vi "M Water Cells 90.vi"(11 "EV3 in":T1) -> (3 "EV3 out":T1)   [LabVIEW 2016]
uses:
  <vilib>/NXT/Subs/LVHSConnector.ctl
  <vilib>/NXT/LegoClasses/BrickReference/BrickReference.lvclass
  <vilib>/NXT/Dual Mode Library/Waits/Wait_Num.vi
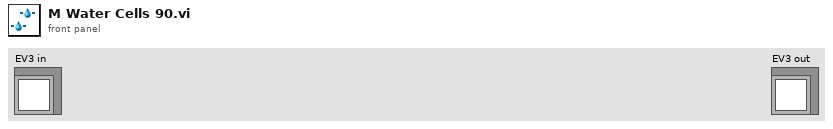
[diagram p1: front panel]
types:
  T1 = typedef "LVHSConnector.ctl" = refnum<class "BrickReference.lvclass">
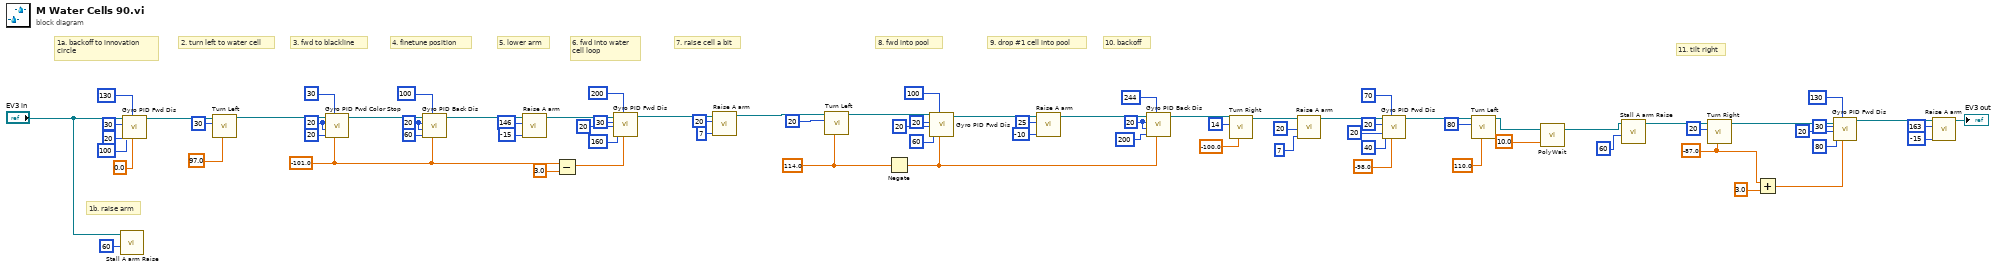
[diagram p0: block diagram]
diagram:
  w34 = sgl 114.0 ("Turning angle")
  w24 = sgl -87.0 ("Turning angle")
  w44 = 20 ("Max. speed")
  w63 = 20 ("Max. speed")
  w41 = sgl -101.0 ("Target angle")
  w67 = 20 ("Max. speed")
  # "11. tilt right"
  # "10. backoff"
  # "8. fwd into pool"
  # "6. fwd into water\ncell loop"
  # "4. finetune position"
  # "3. fwd to blackline"
  # "1b. raise arm"
  # "9. drop #1 cell into pool"
  # "7. raise cell a bit"
  # "5. lower arm"
  # "2. turn left to water cell"
  # "1a. backoff to innovation\ncircle"
  n1 = call "Stall A arm Raise.vi"("Power"=i8 60, "NXT/EV3"="EV3 in") -> ()  [unwired: 9 in, 1 out]
  n2 = call "Gyro PID Fwd Dis.vi"("Target angle"=sgl 0.0, "Threshold to stop"=130, "Threshold to slow"=100, "Min. speed"=20, "Max. speed"=30, "EV3 in"="EV3 in") -> ("EV3 out"=w76:T1)  [unwired: 5 in]
  n3 = call "Turn Left.vi"("Turning angle"=sgl 97.0, "Motor B (right)"=i8 30, "EV3 in"=w76) -> ("EV3 out"=w69:T1)  [unwired: 8 in]
  n4 = call "Gyro PID Fwd Color Stop.vi"("Target angle"=w41, "Threshold to Color"=30, "Threshold to slow"=20, "Min. speed"=w67, "Max. speed"=w67, "EV3 in"=w69) -> ("EV3 out"=w65:T1)  [unwired: 5 in]
  n5 = call "Gyro PID Back Dis.vi"("Target angle"=w41, "Threshold to stop"=100, "Threshold to slow"=60, "Min. speed"=w63, "Max. speed"=w63, "EV3 in"=w65) -> ("EV3 out"=w61:T1)  [unwired: 5 in]
  n6 = call "Raise A arm.vi"("Power"=i8 -15, "Rotation"=146, "EV3 in"=w61) -> ("EV3 out"=w60:T1)  [unwired: 8 in]
  n7 = Subtract(x=w41, y=sgl 3.0) -> (x-y=w39:sgl)
  n8 = call "Gyro PID Fwd Dis.vi"("Target angle"=w39, "Threshold to stop"=200, "Threshold to slow"=160, "Min. speed"=20, "Max. speed"=30, "EV3 in"=w60) -> ("EV3 out"=w55:T1)  [unwired: 5 in]
  n9 = call "Raise A arm.vi"("Power"=i8 7, "Rotation"=20, "EV3 in"=w55) -> ("EV3 out"=w37:T1)  [unwired: 8 in]
  n10 = call "Turn Left.vi"("Turning angle"=w34, "Motor B (right)"=i8 20, "EV3 in"=w37) -> ("EV3 out"=w36:T1)  [unwired: 8 in]
  n11 = Negate(x=w34) -> (-x=w33:sgl)
  n12 = call "Gyro PID Fwd Dis.vi"("Target angle"=w33, "Threshold to stop"=100, "Threshold to slow"=60, "Min. speed"=20, "Max. speed"=20, "EV3 in"=w36) -> ("EV3 out"=w47:T1)  [unwired: 5 in]
  n13 = call "Raise A arm.vi"("Power"=i8 -10, "Rotation"=25, "EV3 in"=w47) -> ("EV3 out"=w42:T1)  [unwired: 8 in]
  n14 = call "Gyro PID Back Dis.vi"("Target angle"=w33, "Threshold to stop"=244, "Threshold to slow"=200, "Min. speed"=w44, "Max. speed"=w44, "EV3 in"=w42) -> ("EV3 out"=w15:T1)  [unwired: 5 in]
  n15 = call "Turn Right.vi"("Turning angle"=sgl -100.0, "Motor B (right)"=i8 14, "EV3 in"=w15) -> ("EV3 out"=w13:T1)  [unwired: 8 in]
  n16 = call "Raise A arm.vi"("Power"=i8 7, "Rotation"=20, "EV3 in"=w13) -> ("EV3 out"=w8:T1)  [unwired: 8 in]
  n17 = call "Gyro PID Fwd Dis.vi"("Target angle"=sgl -98.0, "Threshold to stop"=70, "Threshold to slow"=40, "Min. speed"=20, "Max. speed"=20, "EV3 in"=w8) -> ("EV3 out"=w7:T1)  [unwired: 5 in]
  n18 = call "Turn Left.vi"("Turning angle"=sgl 110.0, "Motor B (right)"=i8 80, "EV3 in"=w7) -> ("EV3 out"=w1:T1)  [unwired: 8 in]
  n19 = call-poly <vilib>:"PolyWait.vi"("Time (1 sec)"=sgl 10.0, "NXT/EV3"=w1) -> ("NXT/EV3"=w2:T1)  [unwired: 2 in]
  n20 = call "Stall A arm Raise.vi"("Power"=i8 60, "NXT/EV3"=w2) -> ("NXT/EV3"=w32:T1)  [unwired: 9 in]
  n21 = call "Turn Right.vi"("Turning angle"=w24, "Motor B (right)"=i8 20, "EV3 in"=w32) -> ("EV3 out"=w26:T1)  [unwired: 8 in]
  n22 = Add(x=w24, y=sgl 3.0) -> (x+y=w23:sgl)
  n23 = call "Gyro PID Fwd Dis.vi"("Target angle"=w23, "Threshold to stop"=130, "Threshold to slow"=80, "Min. speed"=20, "Max. speed"=30, "EV3 in"=w26) -> ("EV3 out"=w22:T1)  [unwired: 5 in]
  n24 = call "Raise A arm.vi"("Power"=i8 -15, "Rotation"=163, "EV3 in"=w22) -> ("EV3 out"=→"EV3 out":T1)  [unwired: 8 in]
